vi "close ASI stage.vi"(8 "error in (no error)":errorcluster, 11 "ASI stage":T1) -> (0 "error out":errorcluster)   [LabVIEW 2010]
uses:
  stage properties.ctl
  <vilib>/Instr/_visa.llb/VISA Flush IO Buffer Mask.ctl
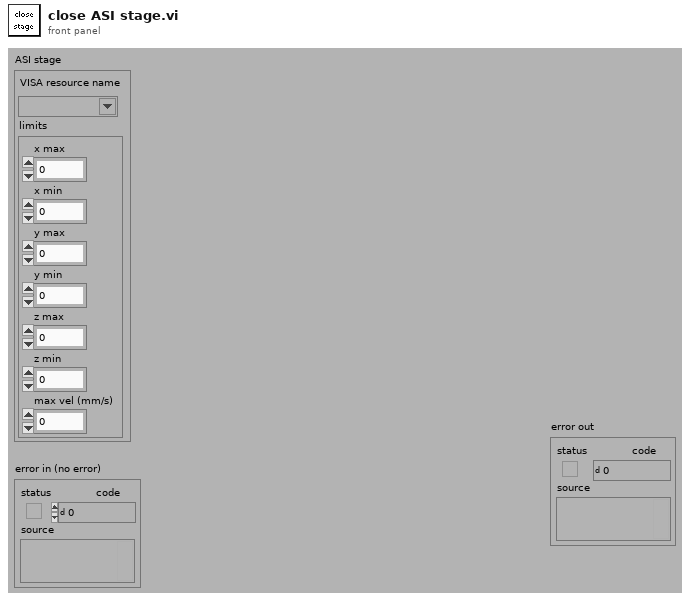
[diagram p1: front panel]
types:
  T1 = typedef "stage properties.ctl" = cluster{"VISA resource name":refnum<visa-resource-name>, "limits":cluster{"x max":dbl, "x min":dbl, "y max":dbl, "y min":dbl, "z max":dbl, "z min":dbl, "max vel (mm/s)":dbl}}
  T2 = typedef "VISA Flush IO Buffer Mask.ctl" = u16
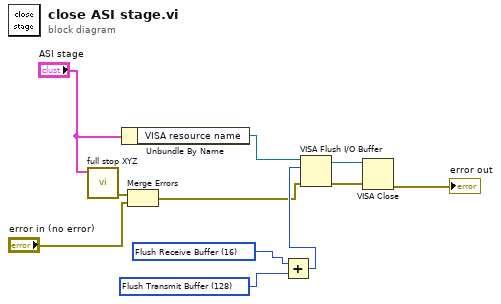
[diagram p0: block diagram]
diagram:
  w11 = T2 128 items=["Flush Receive Buffer"=16, "Write Transmit Buffer to Device"=32, "Flush Receive Buffer (No I/O)"=64, "Flush Transmit Buffer"=128] ("Mask")
  w10 = T2 16 items=["Flush Receive Buffer"=16, "Write Transmit Buffer to Device"=32, "Flush Receive Buffer (No I/O)"=64, "Flush Transmit Buffer"=128] ("Mask")
  n1 = call "full stop XYZ.vi"("ASI stage"="ASI stage") -> ("error out"=w7:errorcluster)  [unwired: 10 in]
  n2 = Unbundle By Name("ASI stage") -> ("VISA resource name"=w6:refnum<visa-resource-name>)
  n3 = Merge Errors(w7, "error in (no error)") -> (w2:errorcluster)
  n4 = Add(x=w10, y=w11) -> (x+y=w9:T2)
  n5 = VISA Flush I/O Buffer(VISA resource name=w6, mask (16)=w9, error in (no error)=w2) -> (VISA resource name out=w4:refnum<visa-resource-name>, error out=w5:errorcluster)
  n6 = VISA Close(VISA resource name=w4, error in (no error)=w5) -> (error out=→"error out":errorcluster)
